vi "7HP_EnFlo_Specific - USB.vi"(2 "Datalog file path (full)":path, 3 "COM port":refnum<visa-resource-name>, 4 "Log data stream":bool, 5 "Data rate (Hz)":u8(ring)=14 items=["1", "2", "4", "5", "8", "10", "16", "20", "25", "32", "40", "50", "64", "80", "100", "125", "160", "200", "250", "320", "400", "500", "625", "800", "1000"], 6 "N samples":u32=1000, 7 "Command":T2="s") -> (0 "Error":errorcluster, 1 "All samples out":sgl[][](array[numeric]))   [LabVIEW 2017]
uses:
  ctls/Cmd (USB).ctl
panel:
  in  "Main":T1(tab)
  out "Serial number":u32 format="%08x"
  out "Pressure sensor EEPROM checksums ok":bool[](array[boolean])
  out "Pressure sensor temperatures in range":bool[](array[boolean])
  out "Pressure sensor values in range":bool[](array[boolean])
  out "Subsystems ok":bool[](array[boolean])
  out "n":u16
  out "Auto zero progBar":u16(slide) caption="Collecting samples, please maintain dP = 0" scale=0.0..1000.0
  out "P_raw_Azero":sgl[](array[numeric])
  out "Chk ok":bool
  out "EEPROM Checksum":u8 format="%02x"
  in  "EEPROM array":sgl[](array[numeric])
  out "sent":bool
  in  "Stop Data":bool
  out "Relative humidity (%)":sgl
  out "Env. sensor die temperature (deg C)":sgl
  out "External thermistor temperature (deg C)":sgl
  out "Atmospheric pressure (mbar)":sgl
  out "Checksum ok":bool
  out "Gyration vector (deg / s)":sgl[](array[numeric])
  out "Acceleration vector (g)":sgl[](array[numeric])
  out "Pressures":sgl[][](graph)
  out "Stream enabled":bool
  # "Paul Nathan 10/2017"
  # "Output array order:\nP0.... (Pa)\n.\n.\nP6.... (Pa)\nP_atmos (mbar)....\nT_ext (deg C)....\nT_env (deg C)....\nRH (%)....\nax (g)....\nay (g)....\naz (g)....\nwx (deg / s)....\nwy (deg / s)....\nwz (deg / s)...."
  # "Pressure sensor 0 EEPROM checksum okay"
  # "Pressure sensor 1 EEPROM checksum okay"
  # "Pressure sensor 2 EEPROM checksum okay"
  # "Pressure sensor 3 EEPROM checksum okay"
  # "Pressure sensor 4 EEPROM checksum okay"
  # "Pressure sensor 5 EEPROM checksum okay"
  # "Pressure sensor 6 EEPROM checksum okay"
  # "Pressure sensor 0 temperature in range"
  # "Pressure sensor 1 temperature in range"
  # "Pressure sensor 2 temperature in range"
  # "Pressure sensor 3 temperature in range"
  # "Pressure sensor 4 temperature in range"
  # "Pressure sensor 5 temperature in range"
  # "Pressure sensor 6 temperature in range"
  # "Pressure sensor 0 value in range"
  # "Pressure sensor 1 value in range"
  # "Pressure sensor 2 value in range"
  # "Pressure sensor 3 value in range"
  # "Pressure sensor 4 value in range"
  # "Pressure sensor 5 value in range"
  # "Pressure sensor 6 value in range"
  # "Environmental sensor present"
  # "Inertial sensor present"
  # "Accelerometer self test pass"
  # "Gyroscope self test pass"
  # "External thermistor value in range"
  # "MCU EEPROM checksum ok"
  # "of 1000"
  # "P0 raw auto-zero"
  # "P1 raw auto-zero"
  # "P2 raw auto-zero"
  # "P3 raw auto-zero"
  # "P4 raw auto-zero"
  # "P5 raw auto-zero"
  # "P6 raw auto-zero"
  # "P0 raw auto-zero"
  # "P1 raw auto-zero"
  # "P2 raw auto-zero"
  # "P3 raw auto-zero"
  # "P4 raw auto-zero"
  # "P5 raw auto-zero"
  # "P6 raw auto-zero"
  # "Atmospheric pressure offset (Pa)"
  # "External thermistor temperature offset (deg C)"
  # "Serial number"
  # "(reserved, 0x00000000)"
  # "Accelerometer vector magnitude scale factor"
  # "(reserved, 0x00000000)"
  # "(reserved, 0x00000000)"
  # "Gyroscope x component offset (deg / s)"
  # "Gyroscope y component offset (deg / s)"
  # "Gyroscope z component offset (deg / s)"
  # "w_x"
  # "w_y"
  # "w_z"
  # "a_x"
  # "a_y"
  # "a_z"
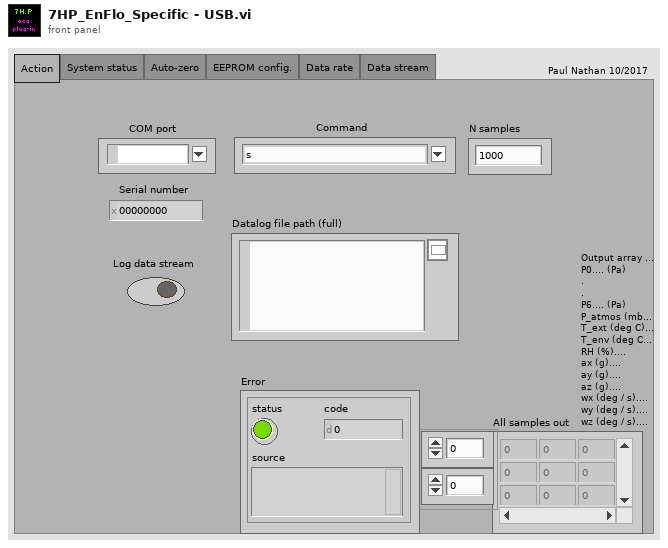
[diagram p1: front panel]
types:
  T1 = enum32{"Action", "System status", "Auto-zero", "EEPROM config.", "Data rate", "Data stream"}
  T2 = typedef "Cmd (USB).ctl" = string
  T3 = enum16{"open", "replace", "create", "open or create", "replace or create", "replace or create with confirmation"}
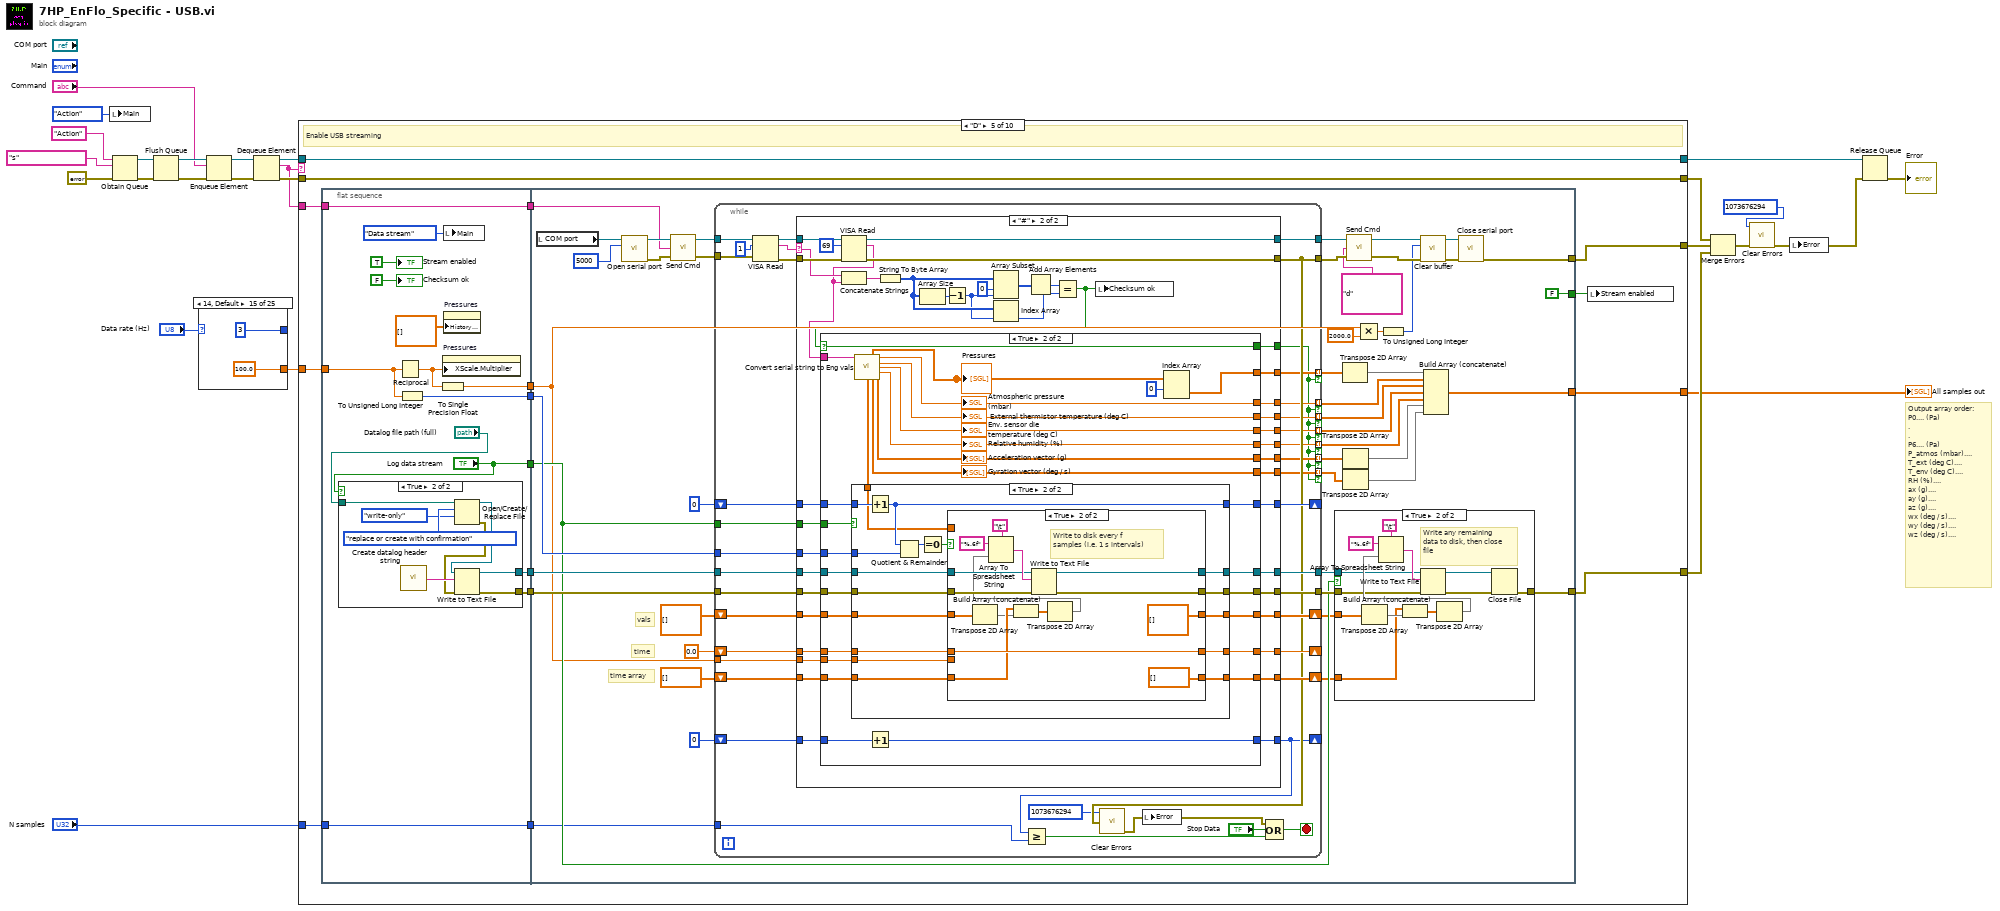
[diagram p0: block diagram]
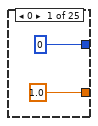
[diagram p2: hidden frame]
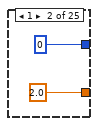
[diagram p3: hidden frame]
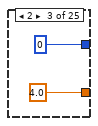
[diagram p4: hidden frame]
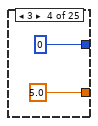
[diagram p5: hidden frame]
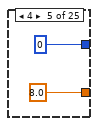
[diagram p6: hidden frame]
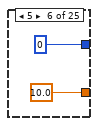
[diagram p7: hidden frame]
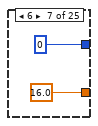
[diagram p8: hidden frame]
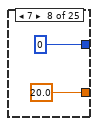
[diagram p9: hidden frame]
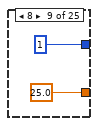
[diagram p10: hidden frame]
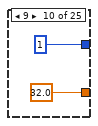
[diagram p11: hidden frame]
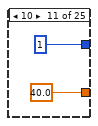
[diagram p12: hidden frame]
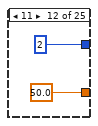
[diagram p13: hidden frame]
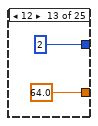
[diagram p14: hidden frame]
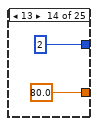
[diagram p15: hidden frame]
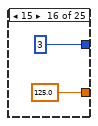
[diagram p16: hidden frame]
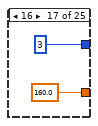
[diagram p17: hidden frame]
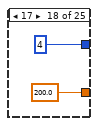
[diagram p18: hidden frame]
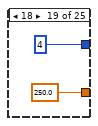
[diagram p19: hidden frame]
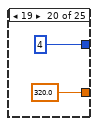
[diagram p20: hidden frame]
diagram:
  # "Output array order:\nP0.... (Pa)\n.\n.\nP6.... (Pa)\nP_atmos (mbar)....\nT_ext (deg C)....\nT_env (deg C)....\nRH (%)....\nax (g)....\nay (g)....\naz (g)....\nwx (deg / s)....\nwy (deg / s)....\nwz (deg / s)...."
  n1 = local write "Main"(T1."Action" ("Main")) -> ()
  n2 = Obtain Queue(name (unnamed)="Action", element data type=T2 "s" ("Combo Box"), error in (no error)=errorcluster {"status"=FALSE, "code"=0, "source"=""}) -> (queue out=w24:refnum<queue>, error out=w25:errorcluster)  [unwired: 2 in, 1 out]
  n3 = Flush Queue(queue=w24, error in (no error)=w25) -> (queue out=w22:refnum<queue>, error out=w17:errorcluster)  [unwired: 1 out]
  n4 = case shown="14, Default" "Data rate (Hz)" {
    tunnel: [1.0 2.0 4.0 5.0 8.0 10.0 16.0 20.0 25.0 32.0 40.0 50.0 64.0 80.0 100.0 125.0 160.0 200.0 250.0 320.0 400.0 500.0 625.0 800.0 1000.0] -> w2
    tunnel: [u8 0 u8 0 u8 0 u8 0 u8 0 u8 0 u8 0 u8 0 u8 1 u8 1 u8 1 u8 2 u8 2 u8 2 u8 3 u8 3 u8 3 u8 4 u8 4 u8 4 u8 5 u8 5 u8 6 u8 6 u8 6] -> _
    frame 0 {
    }
    frame 1 {
    }
    frame 2 {
    }
    frame 3 {
    }
    frame 4 {
    }
    frame 5 {
    }
    frame 6 {
    }
    frame 7 {
    }
    frame 8 {
    }
    frame 9 {
    }
    frame 10 {
    }
    frame 11 {
    }
    frame 12 {
    }
    frame 13 {
    }
    frame 14, Default {
    }
    frame 15 {
    }
    frame 16 {
    }
    frame 17 {
    }
    frame 18 {
    }
    frame 19 {
    }
    frame 20 {
    }
    frame 21 {
    }
    frame 22 {
    }
    frame 23 {
    }
    frame 24 {
    }
  }
  n5 = Enqueue Element(queue=w22, element="Command", error in (no error)=w17) -> (queue out=w18:refnum<queue>, error out=w16:errorcluster)  [unwired: 1 in, 1 out]
  n6 = Dequeue Element(queue=w18, error in (no error)=w16) -> (queue out=w13:refnum<queue>, element=w11:T2, error out=w12:errorcluster)  [unwired: 1 in, 1 out]
  n7 = case shown="\"D\"" w11 {
    tunnel: w13 -> [w81 w119 w155 w195 w244 w507 w530 w613 w634 w637]
    tunnel: [w81 w119 w155 w195 w244 w507 w530 w613 w634 w637] -> w14
    tunnel: w12 -> [w80 w118 w154 w194 w243 w506 w531 w612 w633 w636]
    tunnel: [w80 w118 w154 w194 w243 w506 w531 w612 w633 w636] -> w10
    tunnel: w11 -> [w79 w117 w153 w193 w242 w509 w533 w611 _ _]
    tunnel: [w77 w115 w151 w190 w240 w508 w532 w609 errorcluster {"status"=FALSE, "code"=0, "source"=""} ("Error out") errorcluster {"status"=FALSE, "code"=0, "source"=""} ("Error out")] -> w9
    tunnel: [_ _ _ _ w239 _ _ _ _ _] -> w8
    tunnel: "N samples" -> [_ _ _ _ w232 _ _ _ _ _]
    tunnel: [_ _ _ _ w230 _ _ _ _ _] -> w4
    tunnel: w2 -> [_ _ _ _ w229 w504 _ _ _ _]
    frame "S", "s" {
      # "Perform self-test and retrieve status bytes, Retrieve status bytes"
      n8 = flat-sequence {
        tunnel: w79 -> [w84]
        tunnel: [w84] -> w78
        tunnel: w78 -> [w90]
        tunnel: [w85] -> w77
        frame #0 {
          w83 = bool[] [] ("Pressure sensor EEPROM checksums ok")
          n9 = local write "Main"(T1."System status" ("Main")) -> ()
          "Pressure sensor EEPROM checksums ok" <- w83
          "Pressure sensor temperatures in range" <- w83
          "Pressure sensor values in range" <- w83
          "Subsystems ok" <- w83
        }
        frame #1 {
          w94 = 1 ("length (rest)")
          w102 = u8 0 ("byte count")
          n10 = local read "COM port"() -> (w91:refnum<visa-resource-name>)
          n11 = call "Open serial port.vi"("timeout (ms)"=u32 5000, "VISA resource name"=w91) -> ("Error out"=w112:errorcluster, "VISA resource name out"=w113:refnum<visa-resource-name>)  [unwired: 8 in]
          n12 = call "Send Cmd.vi"("Error In"=w112, "Operation"=w90, "Port"=w113) -> ("Error Out"=w110:errorcluster, "Port out"=w111:refnum<visa-resource-name>)  [unwired: 1 in]
          n13 = VISA Read(VISA resource name=w111, byte count=u32 4, error in (no error)=w110) -> (VISA resource name out=w108:refnum<visa-resource-name>, read buffer=w97:string, error out=w107:errorcluster)  [unwired: 1 out]
          n14 = call "Close serial port.vi"("Error in"=w107, "VISA resource name"=w108) -> ("Error out"=w85:errorcluster)  [unwired: 9 in]
          n15 = String Subset(string=w97, offset (0)=0, length (rest)=w94) -> (substring=w106:string)
          n16 = String Subset(string=w97, offset (0)=1, length (rest)=w94) -> (substring=w105:string)
          n17 = String Subset(string=w97, offset (0)=2 ("length (rest)"), length (rest)=w94) -> (substring=w104:string)
          n18 = String Subset(string=w97, offset (0)=3, length (rest)=w94) -> (substring=w103:string)
          n19 = Type Cast(type=w102, x=w106) -> (*(type *) &x=w101:u8)
          n20 = Type Cast(type=w102, x=w105) -> (*(type *) &x=w100:u8)
          n21 = Type Cast(type=w102, x=w104) -> (*(type *) &x=w99:u8)
          n22 = Type Cast(type=w102, x=w103) -> (*(type *) &x=w98:u8)
          n23 = Number To Boolean Array(number=w101) -> (Boolean array=w89:bool[])
          n24 = Number To Boolean Array(number=w100) -> (Boolean array=w88:bool[])
          n25 = Number To Boolean Array(number=w99) -> (Boolean array=w87:bool[])
          n26 = Number To Boolean Array(number=w98) -> (Boolean array=w86:bool[])
          n27 = local write "Pressure sensor EEPROM checksums ok"(w89) -> ()
          n28 = local write "Pressure sensor temperatures in range"(w88) -> ()
          n29 = local write "Pressure sensor values in range"(w87) -> ()
          n30 = local write "Subsystems ok"(w86) -> ()
        }
      }
    }
    frame "Z", "z" {
      # "Perform permanent auto-zero (write values to EEPROM), Perform temporary auto-zero"
      n31 = flat-sequence {
        tunnel: w117 -> [w123]
        tunnel: [w123] -> w116
        tunnel: w116 -> [w130]
        tunnel: [w126] -> w115
        frame #0 {
          n32 = local write "Main"(T1."Auto-zero" ("Main")) -> ()
          "P_raw_Azero" <- sgl[] [] ("P_raw_Azero")
          "Auto zero progBar" <- u16 0 ("Collecting samples, please maintain dP = 0")
        }
        frame #1 {
          n33 = local read "COM port"() -> (w131:refnum<visa-resource-name>)
          n34 = call "Open serial port.vi"("timeout (ms)"=u32 16000, "VISA resource name"=w131) -> ("Error out"=w137:errorcluster, "VISA resource name out"=w138:refnum<visa-resource-name>)  [unwired: 8 in]
          n35 = call "Send Cmd.vi"("Error In"=w137, "Operation"=w130, "Port"=w138) -> ("Error Out"=w135:errorcluster, "Port out"=w136:refnum<visa-resource-name>)  [unwired: 1 in]
          n36 = VISA Read(VISA resource name=w136, byte count=u32 28, error in (no error)=w135) -> (VISA resource name out=w133:refnum<visa-resource-name>, read buffer=w127:string, error out=w132:errorcluster)  [unwired: 1 out]
          n37 = for {
            N: 1000 -> [_]
            shift-right: [w140] -> _
            shift-left: u16 0 -> [w141]
            n38 = Increment(x=w141) -> (x+1=w140:u16)
            "n" <- w140
            n39 = Wait (ms)(milliseconds to wait=u32 11) -> ()  [unwired: 1 out]
            n40 = local write "Auto zero progBar"(w140) -> ()
          }
          n41 = for {
            N: 7 -> [_]
            tunnel: [w144] -> w129 mode=indexing
            tunnel: w127 -> [w143]
            i -> [w150]
            w148 = 4 ("x")
            # "to BE"
            n42 = Multiply(x=w148, y=w150) -> (x*y=w149:i32)
            n43 = String Subset(string=w143, offset (0)=w149, length (rest)=w148) -> (substring=w147:string)
            n44 = Reverse String(1:w147) -> (0:w146:string)
            n45 = Type Cast(type=sgl 0.0 ("byte count"), x=w146) -> (*(type *) &x=w144:sgl)
          }
          n46 = call "Close serial port.vi"("Error in"=w132, "VISA resource name"=w133) -> ("Error out"=w126:errorcluster)  [unwired: 9 in]
          n47 = local write "P_raw_Azero"(w129) -> ()
        }
      }
    }
    frame "R" {
      # "Read all EEPROM values"
      n48 = flat-sequence {
        tunnel: w153 -> [w158]
        tunnel: [w158] -> w152
        tunnel: w152 -> [w172]
        tunnel: [w159] -> w151
        frame #0 {
          n49 = local write "EEPROM array"(sgl[] [] ("EEPROM array")) -> ()
          n50 = local write "Main"(T1."EEPROM config." ("Main")) -> ()
        }
        frame #1 {
          n51 = local read "COM port"() -> (w173:refnum<visa-resource-name>)
          n52 = call "Open serial port.vi"("timeout (ms)"=u32 5000, "VISA resource name"=w173) -> ("Error out"=w179:errorcluster, "VISA resource name out"=w180:refnum<visa-resource-name>)  [unwired: 8 in]
          n53 = call "Send Cmd.vi"("Error In"=w179, "Operation"=w172, "Port"=w180) -> ("Error Out"=w177:errorcluster, "Port out"=w178:refnum<visa-resource-name>)  [unwired: 1 in]
          n54 = VISA Read(VISA resource name=w178, byte count=u32 70, error in (no error)=w177) -> (VISA resource name out=w175:refnum<visa-resource-name>, read buffer=w168:string, error out=w174:errorcluster)  [unwired: 1 out]
          n55 = String To Byte Array(string=w168) -> (unsigned byte array=w162:u8[])
          n56 = call "Close serial port.vi"("Error in"=w174, "VISA resource name"=w175) -> ("Error out"=w159:errorcluster)  [unwired: 9 in]
          n57 = for {
            N: 17 -> [_]
            tunnel: [w185] -> w170 mode=indexing
            tunnel: w168 -> [w184]
            i -> [w189]
            w187 = 4 ("x")
            # "to BE"
            n58 = Multiply(x=w187, y=w189) -> (x*y=w188:i32)
            n59 = String Subset(string=w184, offset (0)=w188, length (rest)=w187) -> (substring=w183:string)
            n60 = Reverse String(1:w183) -> (0:w182:string)
            n61 = Type Cast(type=sgl 0.0 ("byte count"), x=w182) -> (*(type *) &x=w185:sgl)
          }
          n62 = Array Size(array=w162) -> (size(s)=w164:i32)
          n63 = Decrement(x=w164) -> (x-1=w163:i32)
          n64 = Index Array(array=w162, index=69) -> (element=w166:u8)
          n65 = Array Subset(array=w162, index=0, length=w163) -> (w160:u8[])
          n66 = Add Array Elements(numeric array=w160) -> (sum=w161:u8)
          n67 = Equal?(x=w166, y=w161) -> (x = y?=w169:bool)
          n68 = local write "EEPROM array"(w170) -> ()
          n69 = local write "EEPROM Checksum"(w166) -> ()
          n70 = local write "Chk ok"(w169) -> ()
        }
      }
    }
    frame "W" {
      # "Write all EEPROM values (including new checksum)"
      n71 = flat-sequence {
        tunnel: w193 -> [w198]
        tunnel: [w198] -> w192
        tunnel: ["EEPROM array"] -> w191
        tunnel: w192 -> [w214]
        tunnel: w191 -> [w207]
        tunnel: [w205] -> w190
        frame #0 {
          n72 = local write "Main"(T1."EEPROM config." ("Main")) -> ()
        }
        frame #1 {
          n73 = local read "COM port"() -> (w215:refnum<visa-resource-name>)
          n74 = for {
            N: 17 -> [_]
            tunnel: w207 -> [w225] mode=indexing
            shift-right: [w226] -> w200
            shift-left: "" -> [w227]
            # "to LE"
            n75 = Type Cast(type="", x=w225) -> (*(type *) &x=w224:string)
            n76 = Reverse String(1:w224) -> (0:w223:string)
            n77 = Concatenate Strings(w227, w223) -> (w226:string)
          }
          n78 = call "Open serial port.vi"("timeout (ms)"=u32 5000, "VISA resource name"=w215) -> ("Error out"=w220:errorcluster, "VISA resource name out"=w221:refnum<visa-resource-name>)  [unwired: 8 in]
          n79 = call "Send Cmd.vi"("Error In"=w220, "Operation"=w214, "Port"=w221) -> ("Error Out"=w218:errorcluster, "Port out"=w219:refnum<visa-resource-name>)  [unwired: 1 in]
          n80 = Type Cast(type="", x=u8 0) -> (*(type *) &x=w201:string)
          n81 = Concatenate Strings(w200, w201) -> (w199:string)
          n82 = String To Byte Array(string=w199) -> (unsigned byte array=w204:u8[])
          n83 = Add Array Elements(numeric array=w204) -> (sum=w206:u8)
          "EEPROM Checksum" <- w206
          n84 = Type Cast(type="", x=w206) -> (*(type *) &x=w210:string)
          n85 = Concatenate Strings(w199, w210) -> (w209:string)
          n86 = VISA Write(VISA resource name=w219, write buffer=w209, error in (no error)=w218) -> (VISA resource name out=w217:refnum<visa-resource-name>, error out=w216:errorcluster)  [unwired: 1 out]
          n87 = call "Close serial port.vi"("Error in"=w216, "VISA resource name"=w217) -> ("Error out"=w205:errorcluster)  [unwired: 9 in]
          "Chk ok" <- TRUE ("Chk ok")
        }
      }
    }
    frame "D" {
      # "Enable USB streaming"
      n88 = flat-sequence {
        tunnel: w242 -> [w258]
        tunnel: [w258] -> w241
        tunnel: [w255] -> w238
        tunnel: [w254] -> w237
        tunnel: [w252] -> w236
        tunnel: w229 -> [w253]
        tunnel: [w250] -> w235
        tunnel: ["Log data stream"] -> w234
        tunnel: w232 -> [w246]
        tunnel: [w246] -> w231
        tunnel: w241 -> [w297]
        tunnel: [w312] -> w240
        tunnel: [w311] -> w239
        tunnel: w238 -> [w308]
        tunnel: w237 -> [w307]
        tunnel: w236 -> [w309]
        tunnel: w235 -> [w286]
        tunnel: w234 -> [w301]
        tunnel: [FALSE] -> w233
        tunnel: w231 -> [w280]
        tunnel: [w269] -> w230
        frame #0 {
          n89 = case shown="True" "Log data stream" {
            tunnel: "Datalog file path (full)" -> [_ w268]
            tunnel: [refnum<file> refnum ("refnum out") w262] -> w255
            tunnel: [errorcluster {"status"=FALSE, "code"=0, "source"=""} ("error out") w261] -> w254
            frame False {
            }
            frame True {
              n90 = call "Create datalog header string.vi"() -> ("Datalog header string"=w264:string)  [unwired: 1 in]
              n91 = Open/Create/Replace File(file path (use dialog)=w268, operation (0:open)=T3."replace or create with confirmation", access (0:read/write)=enum16{"read/write", "read-only", "write-only"}."write-only") -> (refnum out=w265:refnum<file>, error out=w263:errorcluster)  [unwired: 3 in, 1 out]
              n92 = Write to Text File(file (use dialog)=w265, text=w264, error in=w263) -> (refnum out=w262:refnum<file>, error out=w261:errorcluster)  [unwired: 1 in, 1 out]
            }
          }
          n93 = Reciprocal(x=w253) -> (1/x=w251:dbl)
          n94 = To Unsigned Long Integer(number=w253) -> (unsigned 32bit integer=w252:u32)
          n95 = To Single Precision Float(number=w251) -> (single precision float=w250:sgl)
          n96 = property on="Pressures" class="WFChart (strict)"("XScale.Multiplier"=w251) -> ()  [unwired: 2 in, 2 out]
          n97 = local write "Main"(T1."Data stream" ("Main")) -> ()
          n98 = property on="Pressures" class="WFChart (strict)"("History Data"=sgl[][] []) -> ()  [unwired: 2 in, 2 out]
          "Checksum ok" <- FALSE ("Checksum ok")
          "Stream enabled" <- TRUE ("Stream enabled")
        }
        frame #1 {
          # "vals"
          # "time"
          # "time array"
          n99 = local read "COM port"() -> (w313:refnum<visa-resource-name>)
          n100 = call "Open serial port.vi"("timeout (ms)"=u32 5000, "VISA resource name"=w313) -> ("Error out"=w298:errorcluster, "VISA resource name out"=w300:refnum<visa-resource-name>)  [unwired: 8 in]
          n101 = call "Send Cmd.vi"("Error In"=w298, "Operation"=w297, "Port"=w300) -> ("Error Out"=w296:errorcluster, "Port out"=w299:refnum<visa-resource-name>)  [unwired: 1 in]
          n102 = while {
            tunnel: [w343] -> w294
            tunnel: w299 -> [w345]
            tunnel: [w363] -> w295
            shift-right: [w359] -> _
            shift-left: u32 0 -> [w360]
            tunnel: w309 -> [w358]
            tunnel: w308 -> [w357]
            tunnel: w307 -> [w356]
            tunnel: [w355] -> w306
            tunnel: [w354] -> w305
            shift-right: [w353] -> w283
            shift-left: sgl[][] [] -> [w352]
            shift-right: [w349] -> _
            shift-left: sgl 0.0 ("Numeric") -> [w351]
            tunnel: w286 -> [w350]
            shift-right: [w347] -> w282
            shift-left: sgl[] [] -> [w348]
            tunnel: w301 -> [w346]
            tunnel: w296 -> [w344]
            shift-right: [w337] -> _
            shift-left: u32 0 -> [w340]
            tunnel: w280 -> [w339]
            tunnel: [w336] -> w279 mode=indexing if=w329
            tunnel: [w335] -> w275 mode=indexing if=w329
            tunnel: [w334] -> w274 mode=indexing if=w329
            tunnel: [w333] -> w273 mode=indexing if=w329
            tunnel: [w332] -> w272 mode=indexing if=w329
            tunnel: [w331] -> w277 mode=indexing if=w329
            tunnel: [w330] -> w276 mode=indexing if=w329
            stop <- w361 stop-if-true
            n103 = VISA Read(VISA resource name=w345, byte count=u32 1, error in (no error)=w344) -> (VISA resource name out=w365:refnum<visa-resource-name>, read buffer=w366:string, error out=w364:errorcluster)  [unwired: 1 out]
            n104 = case shown="\"#\"" w366 {
              selector: w366 -> [_ w413]
              tunnel: w365 -> [w376 w417]
              tunnel: [w377 w415] -> w343
              tunnel: w364 -> [w377 w418]
              tunnel: [w376 w416] -> w363
              tunnel: w360 -> [w375 w403]
              tunnel: [w375 w402] -> w359
              tunnel: w358 -> [_ w401]
              tunnel: w357 -> [w374 w400]
              tunnel: w356 -> [w373 w399]
              tunnel: [w373 w398] -> w355
              tunnel: [w374 w397] -> w354
              tunnel: [w372 w396] -> w353
              tunnel: w352 -> [w372 w395]
              tunnel: w351 -> [w371 w394]
              tunnel: w350 -> [_ w393]
              tunnel: [w371 w392] -> w349
              tunnel: w348 -> [w370 w391]
              tunnel: [w370 w390] -> w347
              tunnel: w346 -> [_ w389]
              tunnel: w340 -> [w369 w387]
              tunnel: [w369 w386] -> w337
              tunnel: [_ w385] -> w336
              tunnel: [FALSE w384] -> w329
              tunnel: [_ w383] -> w335
              tunnel: [_ w382] -> w334
              tunnel: [_ w381] -> w333
              tunnel: [_ w380] -> w332
              tunnel: [_ w379] -> w331
              tunnel: [_ w378] -> w330
              frame Default {
              }
              frame "#" {
                n105 = VISA Read(VISA resource name=w417, byte count=u32 69, error in (no error)=w418) -> (VISA resource name out=w416:refnum<visa-resource-name>, read buffer=w404:string, error out=w415:errorcluster)  [unwired: 1 out]
                n106 = Concatenate Strings(w413, w404) -> (w405:string)
                n107 = String To Byte Array(string=w405) -> (unsigned byte array=w408:u8[])
                n108 = Array Size(array=w408) -> (size(s)=w411:i32)
                n109 = Decrement(x=w411) -> (x-1=w407:i32)
                n110 = Array Subset(array=w408, index=0, length=w407) -> (w412:u8[])
                n111 = Index Array(array=w408, index=w407) -> (element=w406:u8)
                n112 = Add Array Elements(numeric array=w412) -> (sum=w409:u8)
                n113 = Equal?(x=w409, y=w406) -> (x = y?=w388:bool)
                n114 = case shown="True" w388 {
                  selector: w388 -> [w419 w433]
                  tunnel: w404 -> [_ w455]
                  tunnel: w403 -> [w426 w454]
                  tunnel: [w426 w453] -> w402
                  tunnel: w401 -> [_ w452]
                  tunnel: w400 -> [w425 w450]
                  tunnel: w399 -> [w424 w449]
                  tunnel: [w424 w448] -> w398
                  tunnel: [w425 w447] -> w397
                  tunnel: w395 -> [w423 w446]
                  tunnel: [w423 w445] -> w396
                  tunnel: w394 -> [w422 w444]
                  tunnel: w393 -> [_ w443]
                  tunnel: [w422 w442] -> w392
                  tunnel: w391 -> [w421 w441]
                  tunnel: [w421 w440] -> w390
                  tunnel: w389 -> [_ w439]
                  tunnel: w387 -> [w420 w438]
                  tunnel: [w420 w437] -> w386
                  tunnel: [_ w434] -> w385
                  tunnel: [w419 w433] -> w384
                  tunnel: [_ w432] -> w383
                  tunnel: [_ w431] -> w382
                  tunnel: [_ w430] -> w381
                  tunnel: [_ w429] -> w380
                  tunnel: [_ w428] -> w379
                  tunnel: [_ w427] -> w378
                  frame False {
                  }
                  frame True {
                    n115 = call "Convert serial string to Eng vals.vi"("Serial buffer string (excluding FrameChar)"=w455) -> ("Pressures"=w436:sgl[][], "Atmospheric pressure (mbar)"=w432:sgl, "External thermistor temperature (deg C)"=w431:sgl, "Env. sensor die temperature (deg C)"=w430:sgl, "Relative humidity (%)"=w429:sgl, "All vals"=w451:sgl[], "Gyration vector (deg / s)"=w427:sgl[], "Acceleration vector (g)"=w428:sgl[])  [unwired: 7 in]
                    "Pressures" <- w436
                    "Acceleration vector (g)" <- w428
                    "Gyration vector (deg / s)" <- w427
                    "Atmospheric pressure (mbar)" <- w432
                    "External thermistor temperature (deg C)" <- w431
                    "Env. sensor die temperature (deg C)" <- w430
                    "Relative humidity (%)" <- w429
                    n116 = case shown="True" w439 {
                      tunnel: w454 -> [w461 w478]
                      tunnel: [w461 w477] -> w453
                      tunnel: w452 -> [_ w476]
                      tunnel: w451 -> [_ w473]
                      tunnel: w450 -> [w459 w472]
                      tunnel: w449 -> [w460 w471]
                      tunnel: [w460 w470] -> w448
                      tunnel: [w459 w469] -> w447
                      tunnel: w446 -> [w458 w468]
                      tunnel: [w458 w467] -> w445
                      tunnel: w444 -> [w457 w466]
                      tunnel: w443 -> [_ w465]
                      tunnel: [w457 w464] -> w442
                      tunnel: w441 -> [w456 w463]
                      tunnel: [w456 w462] -> w440
                      frame False {
                      }
                      frame True {
                        n117 = Increment(x=w478) -> (x+1=w477:u32)
                        n118 = Quotient & Remainder(x=w477, y=w476) -> (x-y*floor(x/y)=w475:u32)  [unwired: 1 out]
                        n119 = Equal To 0?(x=w475) -> (x = 0?=w474:bool)
                        n120 = case shown="True" w474 {
                          tunnel: w473 -> [w486 _]
                          tunnel: w472 -> [w487 w500]
                          tunnel: w471 -> [w488 w499]
                          tunnel: [w488 w498] -> w470
                          tunnel: [w487 w497] -> w469
                          tunnel: w468 -> [w480 w492]
                          tunnel: [w479 sgl[][] []] -> w467
                          tunnel: w466 -> [w481 w495]
                          tunnel: w465 -> [w485 _]
                          tunnel: [w484 w495] -> w464
                          tunnel: w463 -> [w483 w494]
                          tunnel: [w482 sgl[] []] -> w462
                          frame False {
                            n121 = Add(x=w481, y=w485) -> (x+y=w484:sgl)
                            n122 = Build Array (concatenate)(w480, w486) -> (w479:sgl[][])
                            n123 = Build Array (concatenate)(w483, w481) -> (w482:sgl[])
                          }
                          frame True {
                            # "Write to disk every f samples (i.e. 1 s intervals)"
                            n124 = Transpose 2D Array(2D array=w492) -> (transposed array=w491:sgl[][])
                            n125 = Build Array (concatenate)(w494, w491) -> (w490:sgl[][])
                            n126 = Transpose 2D Array(2D array=w490) -> (transposed array=w489:sgl[][])
                            n127 = Array To Spreadsheet String(delimiter (Tab)="\t", array=w489, 3:"%.6f" ("format string")) -> (spreadsheet string=w503:string)
                            n128 = Write to Text File(file (use dialog)=w500, text=w503, error in=w499) -> (refnum out=w497:refnum<file>, error out=w498:errorcluster)  [unwired: 1 in, 1 out]
                          }
                        }
                      }
                    }
                    n129 = Increment(x=w438) -> (x+1=w437:u32)
                    n130 = Index Array(array=w436, index (row)=0) -> (element=w434:sgl[])  [unwired: 1 in]
                  }
                }
                n131 = local write "Checksum ok"(w388) -> ()
              }
            }
            n132 = Greater Or Equal?(x=w337, y=w339) -> (x >= y?=w338:bool)
            n133 = call <vilib>:"Clear Errors.vi"("error in (no error)"=w343, "specific error code to clear (0: all)"=1073676294) -> ("error out"=w342:errorcluster)  [unwired: 4 in, 1 out]
            n134 = local write "Error"(w342) -> ()
            n135 = Compound Arithmetic op=OR(w342, "Stop Data", w338) -> (w361:bool)
          }
          n136 = case shown="True" w301 {
            tunnel: [w315 w328] -> w311
            tunnel: w306 -> [w315 w320]
            tunnel: w305 -> [_ w321]
            tunnel: w283 -> [_ w319]
            tunnel: w282 -> [_ w318]
            frame False {
            }
            frame True {
              # "Write any remaining data to disk, then close file"
              n137 = Transpose 2D Array(2D array=w319) -> (transposed array=w325:sgl[][])
              n138 = Build Array (concatenate)(w318, w325) -> (w326:sgl[][])
              n139 = Transpose 2D Array(2D array=w326) -> (transposed array=w327:sgl[][])
              n140 = Array To Spreadsheet String(delimiter (Tab)="\t", array=w327, 3:"%.6f" ("format string")) -> (spreadsheet string=w322:string)
              n141 = Write to Text File(file (use dialog)=w321, text=w322, error in=w320) -> (refnum out=w317:refnum<file>, error out=w316:errorcluster)  [unwired: 1 in, 1 out]
              n142 = Close File(refnum=w317, error in=w316) -> (error out=w328:errorcluster)  [unwired: 1 out]
            }
          }
          n143 = Transpose 2D Array(2D array=w279) -> (transposed array=w278:sgl[][])
          n144 = Transpose 2D Array(2D array=w277) -> (transposed array=w271:sgl[][])
          n145 = Transpose 2D Array(2D array=w276) -> (transposed array=w270:sgl[][])
          n146 = call "Send Cmd.vi"("Error In"=w294, "Operation"=T2 "d" ("Combo Box"), "Port"=w295) -> ("Error Out"=w290:errorcluster, "Port out"=w291:refnum<visa-resource-name>)  [unwired: 1 in]
          n147 = Multiply(x=w286, y=sgl 2000.0) -> (x*y=w287:sgl)
          n148 = To Unsigned Long Integer(number=w287) -> (unsigned 32bit integer=w284:u32)
          n149 = call "Clear buffer.vi"("Error in"=w290, "dt for timeout (ms)"=w284, "VISA resource name in"=w291) -> ("Error out"=w288:errorcluster, "VISA resource name out"=w289:refnum<visa-resource-name>)  [unwired: 3 in]
          n150 = Build Array (concatenate)(w278, w275, w274, w273, w272, w271, w270) -> (w269:sgl[][])
          n151 = call "Close serial port.vi"("Error in"=w288, "VISA resource name"=w289) -> ("Error out"=w312:errorcluster)  [unwired: 9 in]
        }
      }
      n152 = local write "Stream enabled"(w233) -> ()
    }
    frame "d" {
      # "Disable USB streaming"
      n153 = flat-sequence {
        tunnel: [w517] -> w510
        tunnel: w509 -> [w517]
        tunnel: w504 -> [w512]
        tunnel: [w511] -> w505
        tunnel: w510 -> [w525]
        tunnel: [w524] -> w508
        tunnel: w505 -> [w519]
        frame #0 {
          n154 = disable-structure shown="Disabled" {
            frame Disabled {
              n155 = local write "Main"(T1."Data stream" ("Main")) -> ()
            }
            frame Enabled {
            }
          }
          n156 = Reciprocal(x=w512) -> (1/x=w516:dbl)
          n157 = To Single Precision Float(number=w516) -> (single precision float=w514:sgl)
          n158 = Multiply(x=w514, y=sgl 2000.0) -> (x*y=w515:sgl)
          n159 = To Unsigned Long Integer(number=w515) -> (unsigned 32bit integer=w511:u32)
        }
        frame #1 {
          n160 = local read "COM port"() -> (w526:refnum<visa-resource-name>)
          n161 = call "Open serial port.vi"("timeout (ms)"=u32 5000, "VISA resource name"=w526) -> ("Error out"=w527:errorcluster, "VISA resource name out"=w528:refnum<visa-resource-name>)  [unwired: 8 in]
          n162 = call "Send Cmd.vi"("Error In"=w527, "Operation"=w525, "Port"=w528) -> ("Error Out"=w521:errorcluster, "Port out"=w523:refnum<visa-resource-name>)  [unwired: 1 in]
          n163 = call "Clear buffer.vi"("Error in"=w521, "dt for timeout (ms)"=w519, "VISA resource name in"=w523) -> ("Error out"=w520:errorcluster, "VISA resource name out"=w522:refnum<visa-resource-name>)  [unwired: 3 in]
          n164 = call "Close serial port.vi"("Error in"=w520, "VISA resource name"=w522) -> ("Error out"=w524:errorcluster)  [unwired: 9 in]
        }
      }
    }
    frame "F" {
      # "Set data rate"
      n165 = flat-sequence {
        tunnel: [w538] -> w534
        tunnel: w533 -> [w538]
        tunnel: [w542] -> w535
        tunnel: w534 -> [w540]
        tunnel: w535 -> [w607]
        tunnel: [w607] -> w532
        frame #0 {
          n166 = local write "Main"(T1."Data rate" ("Main")) -> ()
          n167 = local write "sent"(FALSE ("sent")) -> ()
        }
        frame #1 {
          w548 = ""
          # "to LE"
          n168 = local read "Data rate (Hz)"() -> (w539:u8)
          n169 = case shown="14, Default" w539 {
            tunnel: [1.0 2.0 4.0 5.0 8.0 10.0 16.0 20.0 25.0 32.0 40.0 50.0 64.0 80.0 100.0 125.0 160.0 200.0 250.0 320.0 400.0 500.0 625.0 800.0 1000.0] -> w543
            tunnel: [u8 0 u8 0 u8 0 u8 0 u8 0 u8 0 u8 0 u8 0 u8 1 u8 1 u8 1 u8 2 u8 2 u8 2 u8 3 u8 3 u8 3 u8 4 u8 4 u8 4 u8 5 u8 5 u8 6 u8 6 u8 6] -> w550
            frame 0 {
            }
            frame 1 {
            }
            frame 2 {
            }
            frame 3 {
            }
            frame 4 {
            }
            frame 5 {
            }
            frame 6 {
            }
            frame 7 {
            }
            frame 8 {
            }
            frame 9 {
            }
            frame 10 {
            }
            frame 11 {
            }
            frame 12 {
            }
            frame 13 {
            }
            frame 14, Default {
            }
            frame 15 {
            }
            frame 16 {
            }
            frame 17 {
            }
            frame 18 {
            }
            frame 19 {
            }
            frame 20 {
            }
            frame 21 {
            }
            frame 22 {
            }
            frame 23 {
            }
            frame 24 {
            }
          }
          n170 = local read "COM port"() -> (w541:refnum<visa-resource-name>)
          n171 = To Unsigned Word Integer(number=w543) -> (unsigned 16bit integer=w549:u16)
          n172 = Type Cast(type=w548, x=w550) -> (*(type *) &x=w546:string)
          n173 = Type Cast(type=w548, x=w549) -> (*(type *) &x=w547:string)
          n174 = call "Open serial port.vi"("timeout (ms)"=u32 5000, "VISA resource name"=w541) -> ("Error out"=w553:errorcluster, "VISA resource name out"=w552:refnum<visa-resource-name>)  [unwired: 8 in]
          n175 = Reverse String(1:w547) -> (0:w545:string)
          n176 = Concatenate Strings(w546, w545) -> (w544:string)
          n177 = call "Send Cmd + Data.vi"("Error In"=w553, "Data"=w544, "Operation"=w540, "Port"=w552) -> ("Error Out"=w555:errorcluster, "Port out"=w554:refnum<visa-resource-name>)  [unwired: 1 in]
          n178 = call "Close serial port.vi"("Error in"=w555, "VISA resource name"=w554) -> ("Error out"=w542:errorcluster)  [unwired: 9 in]
        }
        frame #2 {
          n179 = Unbundle By Name(w607) -> ("status"=w608:bool)
          n180 = Not(x=w608) -> (.not. x?=→"sent":bool)
        }
      }
    }
    frame "N" {
      # "Get serial number"
      n181 = flat-sequence {
        tunnel: w611 -> [w616]
        tunnel: [w616] -> w610
        tunnel: w610 -> [w622]
        tunnel: [w621] -> w609
        frame #0 {
          n182 = local write "Main"(T1."Action" ("Main")) -> ()
          "Serial number" <- u32 0 ("Numeric")
        }
        frame #1 {
          # "to BE"
          n183 = local read "COM port"() -> (w623:refnum<visa-resource-name>)
          n184 = call "Open serial port.vi"("timeout (ms)"=u32 5000, "VISA resource name"=w623) -> ("Error out"=w629:errorcluster, "VISA resource name out"=w630:refnum<visa-resource-name>)  [unwired: 8 in]
          n185 = call "Send Cmd.vi"("Error In"=w629, "Operation"=w622, "Port"=w630) -> ("Error Out"=w627:errorcluster, "Port out"=w628:refnum<visa-resource-name>)  [unwired: 1 in]
          n186 = VISA Read(VISA resource name=w628, byte count=u32 4, error in (no error)=w627) -> (VISA resource name out=w625:refnum<visa-resource-name>, read buffer=w618:string, error out=w624:errorcluster)  [unwired: 1 out]
          n187 = call "Close serial port.vi"("Error in"=w624, "VISA resource name"=w625) -> ("Error out"=w621:errorcluster)  [unwired: 9 in]
          n188 = Reverse String(1:w618) -> (0:w619:string)
          n189 = Type Cast(type=u32 0 ("byte count"), x=w619) -> (*(type *) &x=w617:u32)
          n190 = local write "Serial number"(w617) -> ()
        }
      }
    }
    frame "X" {
      # "Exit"
    }
    frame Default {
    }
  }
  "All samples out" <- w4
  n191 = Merge Errors(w10, w9, w8) -> (w7:errorcluster)
  n192 = call <vilib>:"Clear Errors.vi"("error in (no error)"=w7, "specific error code to clear (0: all)"=1073676294) -> ("error out"=w15:errorcluster)  [unwired: 4 in, 1 out]
  n193 = local write "Error"(w15) -> ()
  n194 = Release Queue(queue=w14, error in (no error)=w15) -> (error out=→"Error":errorcluster)  [unwired: 1 in, 2 out]
